vi "Write Event Info.vi"(8 "error in (no error)":errorcluster, 10 "Event Info":T1, 11 "UserEventInfo in":refnum<class "UserEventInfo.lvclass">) -> (0 "error out":errorcluster, 3 "UserEventInfo out":refnum<class "UserEventInfo.lvclass">)   [LabVIEW 2019, in "EventRecorder.lvlib" / "UserEventInfo.lvclass"]
uses:
  UserEventInfo.lvclass
  UserEventInfo.lvclass/UserEventInfo.ctl
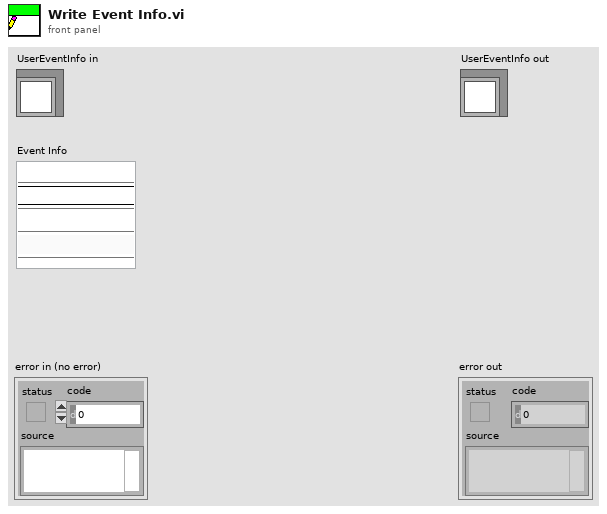
[diagram p1: front panel]
types:
  T1 = cluster{"Event Name":string, "Event Description":string}
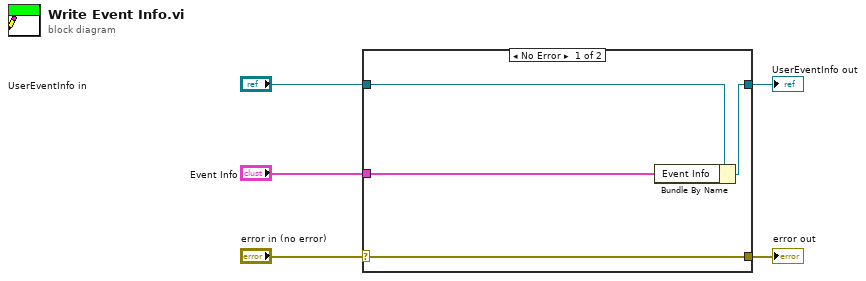
[diagram p0: block diagram]
diagram:
  n1 = case shown="No Error" "error in (no error)" {
    selector: "error in (no error)" -> [w9 w10]
    tunnel: [w9 w10] -> w4
    tunnel: [w7 w11] -> w2
    tunnel: "UserEventInfo in" -> [w8 w11]
    tunnel: "Event Info" -> [w6 _]
    frame No Error {
      n2 = Bundle By Name(cluster=w8, "Event Info"=w6) -> (w7:refnum<class "UserEventInfo.lvclass">)
    }
    frame Error {
    }
  }
  "error out" <- w4
  "UserEventInfo out" <- w2
